vi "State Machine Kernel.vi"(4 "Init?":bool, 5 "Inputs":T4 {"Kobuki Sensors"."Charger Source" items=["DISCHARGING"=0, "DOCKING_CHARGED"=2, "DOCKING_CHARGING"=6, "ADAPTER_CHARGED"=18, "ADAPTER_CHARGING"=22]; "accelerometer"."z axis (g)" format="%.3f"; "accelerometer"."y axis (g)" format="%.3f"; "accelerometer"."x axis (g)" format="%.3f"}, 7 "StateData In":T1) -> (0 "Terminated?":bool, 2 "Outputs":T3, 3 "StateData Out":T1)   [LabVIEW 2017]
uses:
  controls/Inputs.ctl
  shared/Accelerometer.ctl
  Kobuki/KobukiSensors.ctl
  Kobuki/Kobuki Bumps and WheelDrops.ctl
  Kobuki/Kobuki Buttons.ctl
  controls/Outputs.ctl
  controls/StateData.ctl
  controls/StatesEnum.ctl
panel:
  # "Electrical: charging, battery, OI mode"
  # "Sensors: bump, cliff, button, wheel drop"
  # "Motors:"
  # "Inertia"
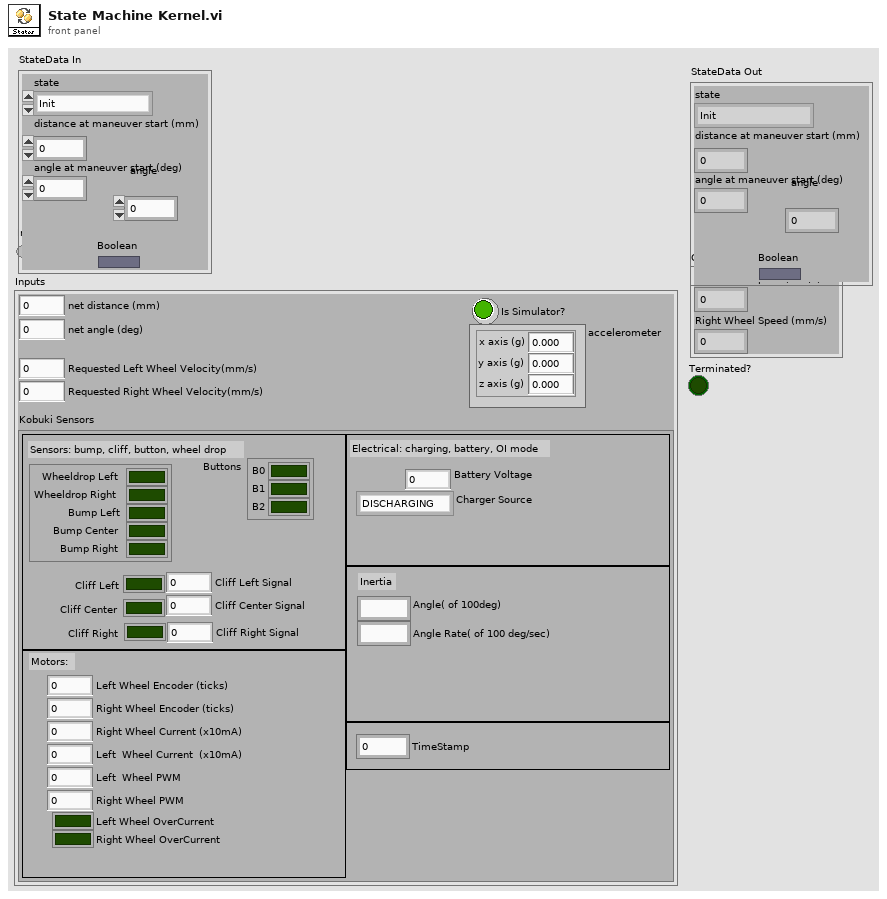
[diagram p1: front panel]
types:
  T1 = typedef "StateData.ctl" = cluster{"distance at maneuver start (mm)":i32, "angle at maneuver start (deg)":i32, "state":T2, "Boolean":bool, "angle":i32}
  T2 = typedef "StatesEnum.ctl" = enum16{"Init", "Center Cliff\n", "Pause", "Drive", "L.Cliff", "R.Cliff", "Shut"}
  T3 = typedef "Outputs.ctl" = cluster{"Left Wheel Speed (mm/s)":i16, "Right Wheel Speed (mm/s)":i16}
  T4 = typedef "Inputs.ctl" = cluster{"net distance (mm)":i32, "net angle (deg)":i32, "accelerometer":T5, "Is Simulator?":bool, "Kobuki Sensors":T6, "Requested Left Wheel Velocity(mm/s)":i32, "Requested Right Wheel Velocity(mm/s)":i32}
  T5 = typedef "Accelerometer.ctl" = cluster{"x axis (g)":dbl, "y axis (g)":dbl, "z axis (g)":dbl}
  T6 = typedef "KobukiSensors.ctl" = cluster{"Bumps + Wheel Drops":T7, "Cliff Left":bool, "Cliff Center":bool, "Cliff Right":bool, "Cliff Left Signal":u16, "Cliff Center Signal":u16, "Cliff Right Signal":u16, "Buttons":T8, "Left Wheel Encoder (ticks)":u16, "Right Wheel Encoder (ticks) ":u16, "Left  Wheel PWM":i8, "Right Wheel PWM":i8, "Left Wheel OverCurrent":bool, "Right Wheel OverCurrent ":bool, "Right Wheel Current (x10mA)":i16, "Left  Wheel Current  (x10mA)":i16, "TimeStamp":u16, "Battery Voltage":dbl, "Angle( of 100deg)":i16, "Angle Rate( of 100 deg/sec)":i16, "Charger Source ":i8}
  T7 = typedef "Kobuki Bumps and WheelDrops.ctl" = cluster{"Wheeldrop Left":bool, "Wheeldrop Right":bool, "Bump Left":bool, "Bump Center":bool, "Bump Right":bool}
  T8 = typedef "Kobuki Buttons.ctl" = cluster{"B0":bool, "B1":bool, "B2":bool}
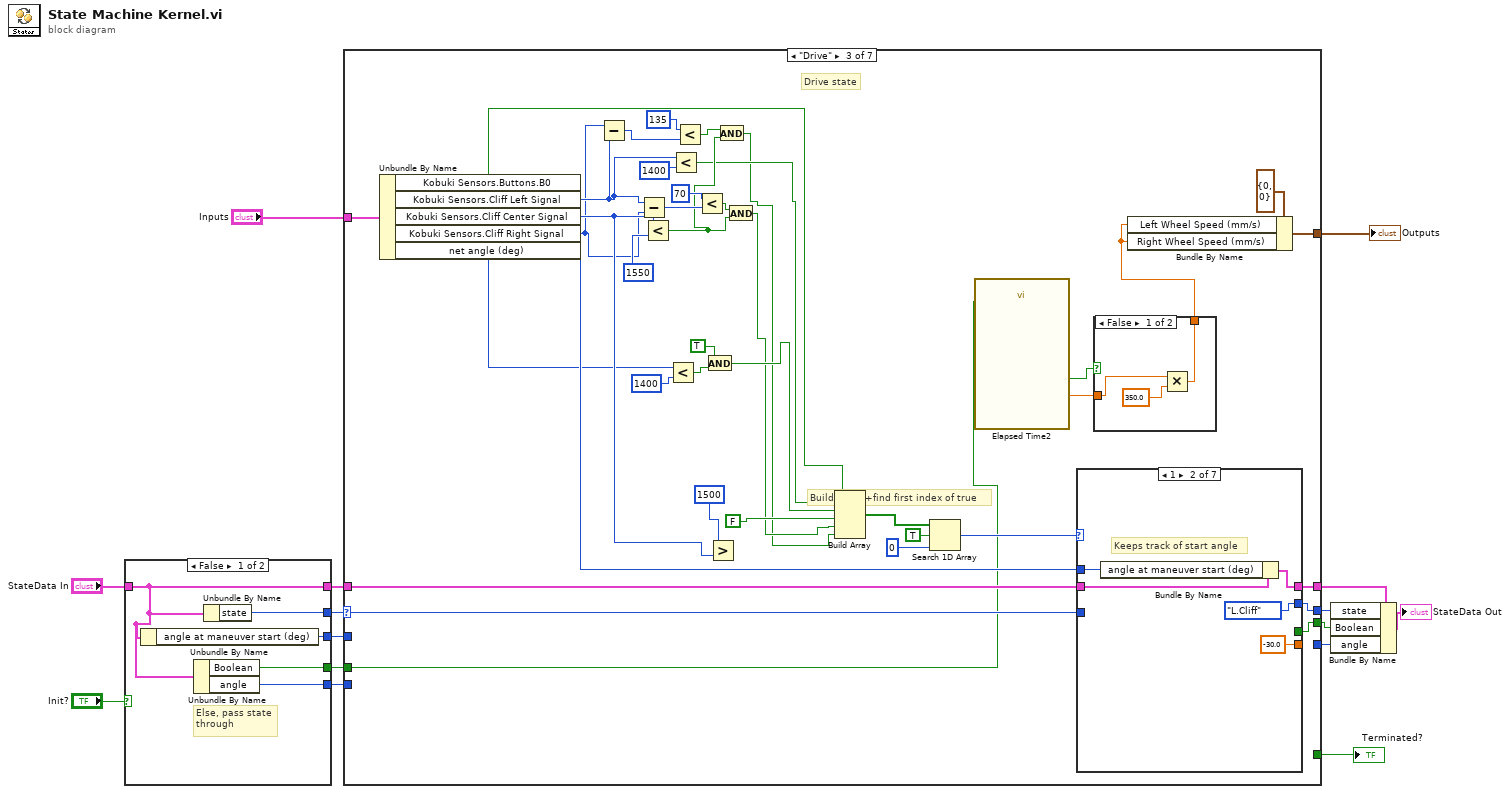
[diagram p0: block diagram]
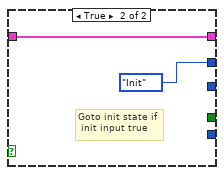
[diagram p2: hidden frame]
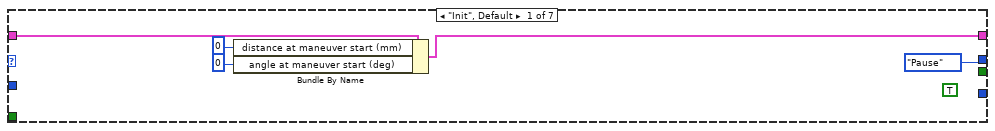
[diagram p3: hidden frame]
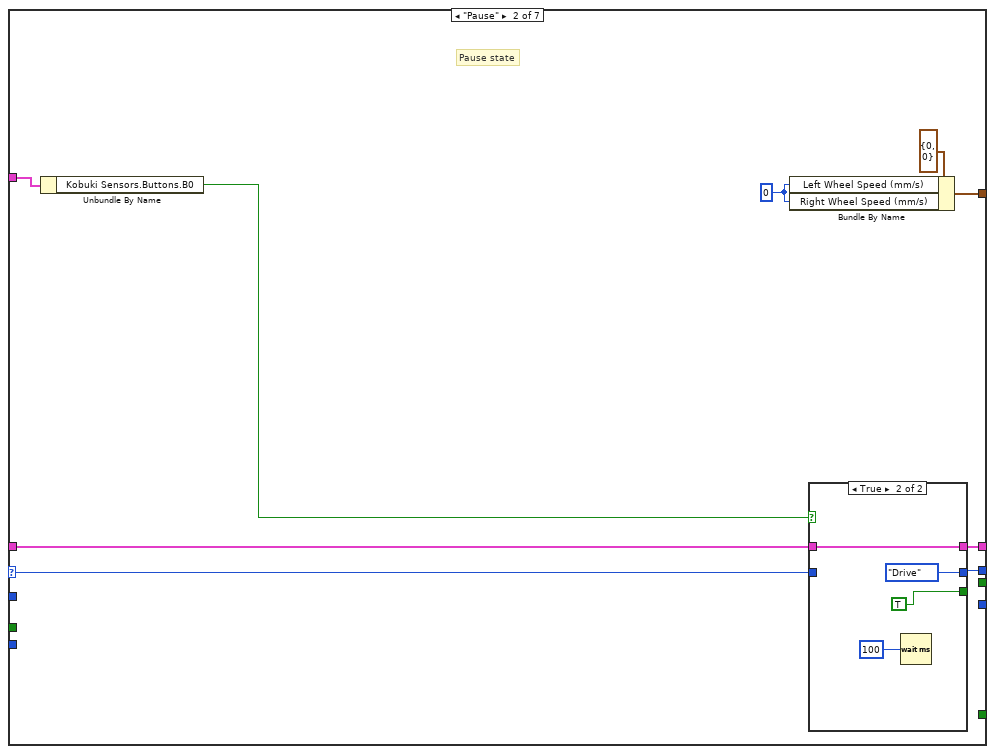
[diagram p4: hidden frame]
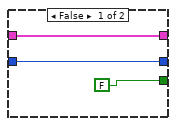
[diagram p5: hidden frame]
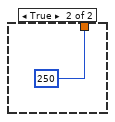
[diagram p6: hidden frame]
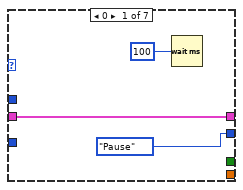
[diagram p7: hidden frame]
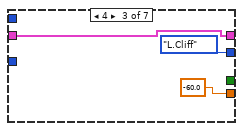
[diagram p8: hidden frame]
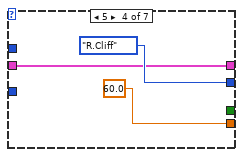
[diagram p9: hidden frame]
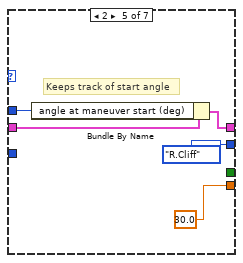
[diagram p10: hidden frame]
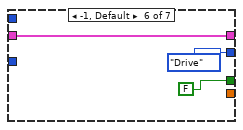
[diagram p11: hidden frame]
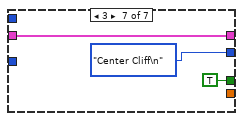
[diagram p12: hidden frame]
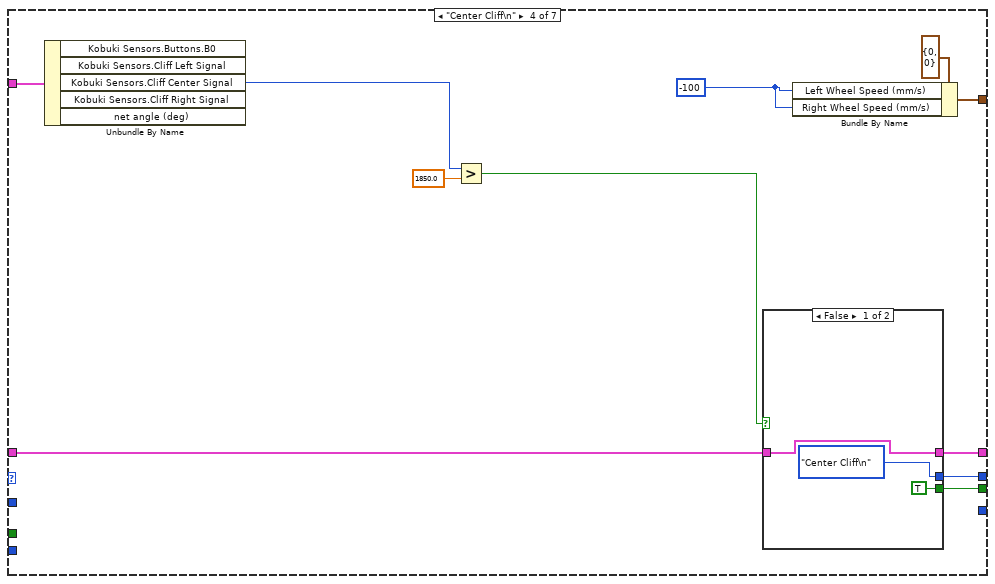
[diagram p13: hidden frame]
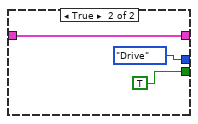
[diagram p14: hidden frame]
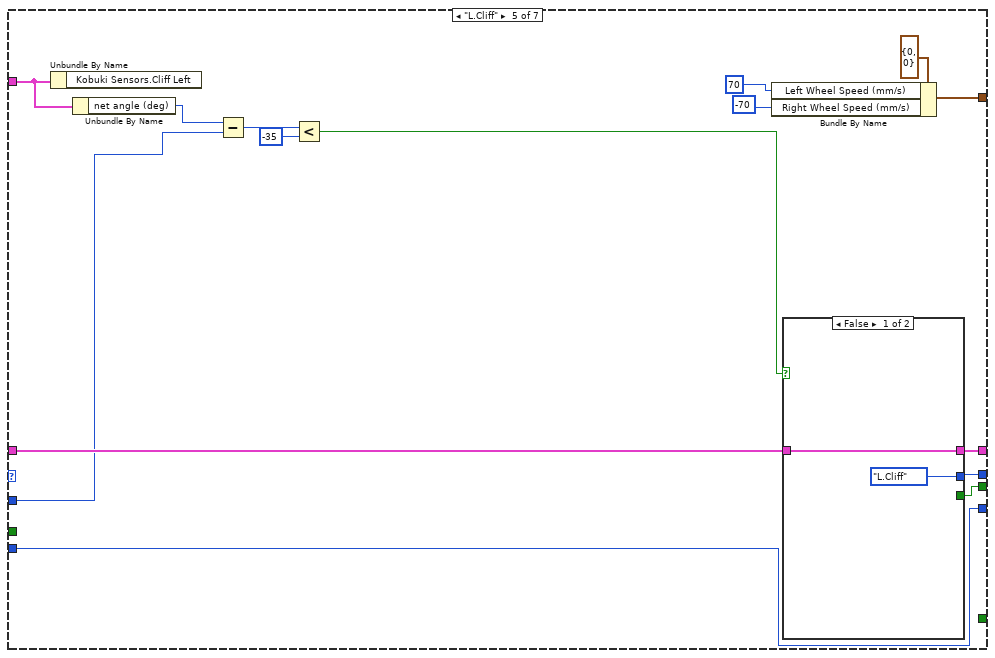
[diagram p15: hidden frame]
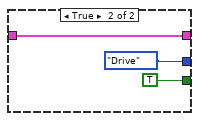
[diagram p16: hidden frame]
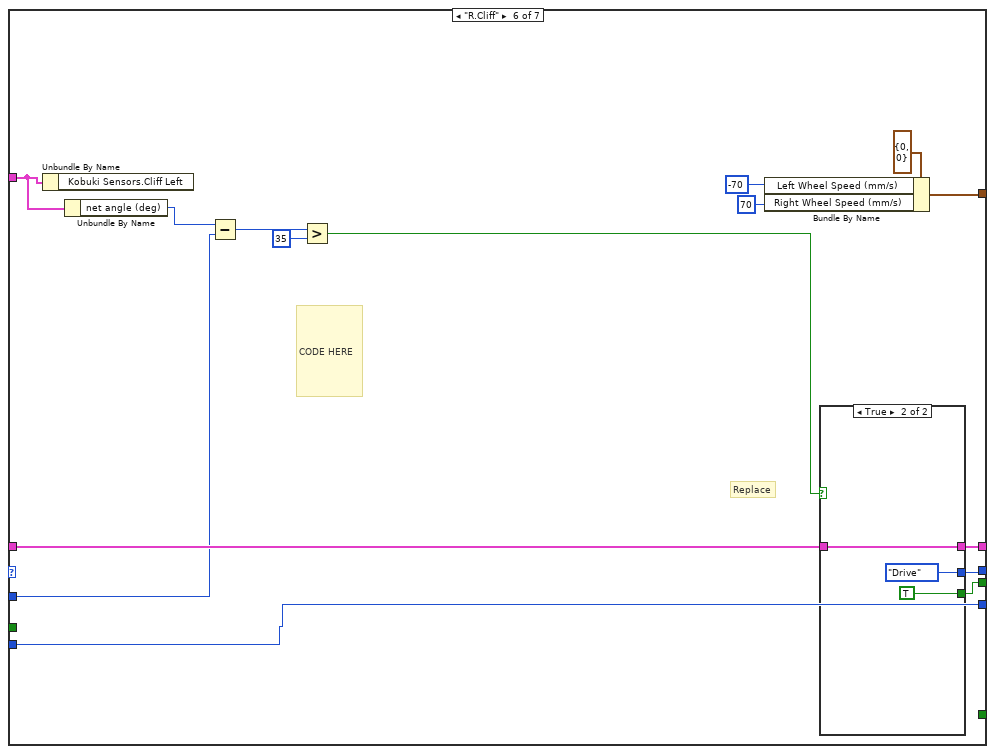
[diagram p17: hidden frame]
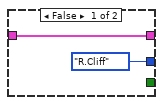
[diagram p18: hidden frame]
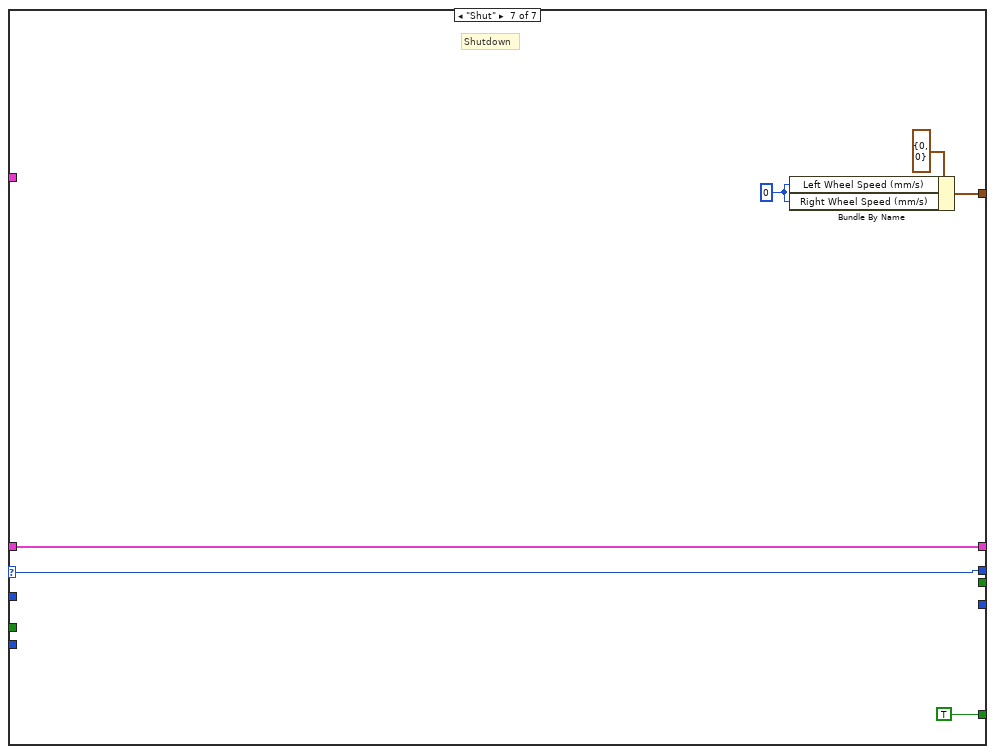
[diagram p19: hidden frame]
diagram:
  n1 = case shown="False" "Init?" {
    tunnel: [w20 StatesEnum."Init" ("StateIn")] -> w13
    tunnel: "StateData In" -> [w18 w21]
    tunnel: [w18 w21] -> w9
    tunnel: [w19 _] -> w6
    tunnel: [w17 _] -> w5
    tunnel: [w16 _] -> w2
    frame False {
      # "Else, pass state \nthrough"
      n2 = Unbundle By Name(w18) -> ("angle at maneuver start (deg)"=w19:i32)
      n3 = Unbundle By Name(w18) -> ("Boolean"=w17:bool, "angle"=w16:i32)
      n4 = Unbundle By Name(w18) -> ("state"=w20:T2)
    }
    frame True {
      # "Goto init state if\n init input true"
    }
  }
  n5 = case shown="\"Drive\"" w13 {
    selector: w13 -> [_ w32 w81 _ _ _ w169]
    tunnel: "Inputs" -> [_ w33 w82 w122 w139 w155 _]
    tunnel: [_ w36 w79 w120 w142 w160 w172] -> w11
    tunnel: [_ _ _ _ _ _ TRUE] -> w12
    tunnel: w9 -> [w27 w30 w74 w118 w140 w158 w170]
    tunnel: [w26 w29 w73 w117 w141 w159 w170] -> w8
    tunnel: w6 -> [_ _ _ _ w137 w154 _]
    tunnel: w5 -> [_ _ w67 _ _ _ _]
    tunnel: [_ _ w60 w116 w131 w151 _] -> w4
    tunnel: [StatesEnum."Pause" ("StateIn") w28 w61 w112 w132 w152 w169] -> w3
    tunnel: w2 -> [_ _ _ _ w130 w150 _]
    tunnel: [_ _ _ _ w130 w150 _] -> w1
    frame "Init", Default {
      (unwired) TRUE
      n6 = Bundle By Name(cluster=w27, "distance at maneuver start (mm)"=0, "angle at maneuver start (deg)"=0) -> (w26:T1)
    }
    frame "Pause" {
      w35 = i16 0 ("Left Wheel Speed (mm/s)")
      # "Pause state"
      n7 = Unbundle By Name(w33) -> ("Kobuki Sensors.Buttons.B0"=w34:bool)
      n8 = Bundle By Name(cluster=T3 {"Left Wheel Speed (mm/s)"=0, "Right Wheel Speed (mm/s)"=0} ("Outputs"), "Left Wheel Speed (mm/s)"=w35, "Right Wheel Speed (mm/s)"=w35) -> (w36:T3)
      n9 = case shown="True" w34 {
        tunnel: w32 -> [w39 _]
        tunnel: [w39 StatesEnum."Drive" ("StateIn")] -> w28
        tunnel: w30 -> [w38 w41]
        tunnel: [w38 w41] -> w29
        tunnel: [FALSE TRUE] -> _
        frame False {
        }
        frame True {
          n10 = Wait (ms)(milliseconds to wait=u32 100) -> ()  [unwired: 1 out]
        }
      }
    }
    frame "Drive" {
      # "Build array +find first index of true"
      # "Drive state"
      n11 = Unbundle By Name(w82) -> ("Kobuki Sensors.Buttons.B0"=w68:bool, "Kobuki Sensors.Cliff Left Signal"=w54:u16, "Kobuki Sensors.Cliff Center Signal"=w59:u16, "Kobuki Sensors.Cliff Right Signal"=w53:u16, "net angle (deg)"=w72:i32)
      n12 = Subtract(x=w53, y=w54) -> (x-y=w52:u16)
      n13 = Subtract(x=w54, y=w53) -> (x-y=w57:u16)
      n14 = Less?(x=w59, y=u16 1550) -> (x < y?=w50:bool)
      n15 = Less?(x=w53, y=u16 1400) -> (x < y?=w69:bool)
      n16 = Less?(x=w54, y=u16 1400) -> (x < y?=w47:bool)
      n17 = Less?(x=u16 135, y=w52) -> (x < y?=w49:bool)
      n18 = Less?(x=u16 70, y=w57) -> (x < y?=w55:bool)
      n19 = And(x=TRUE, y=w69) -> (x .and. y?=w48:bool)
      n20 = Greater?(x=u16 1500 ("y"), y=w59) -> ()  [unwired: 1 out]
      n21 = And(x=w49, y=w50) -> (x .and. y?=w44:bool)
      n22 = And(x=w55, y=w50) -> (x .and. y?=w45:bool)
      n23 = Build Array(w68, w47, w48, FALSE, w45, w44) -> (w78:bool[])
      n24 = Search 1D Array(1D array=w78, element=TRUE, start index (0)=0) -> (index of element=w75:i32)
      n25 = call "Elapsed Time2"("Reset"=w67) -> ("Elapsed Time (s)"=w65:dbl, "Time has Elapsed"=w66:bool)  [unwired: 11 in, 6 out]
      n26 = case shown="1" w75 {
        tunnel: w81 -> [_ _ _ _ _ _ _]
        tunnel: w74 -> [w88 w94 w95 w98 w105 w108 w110]
        tunnel: [w88 w92 w95 w98 w104 w108 w110] -> w73
        tunnel: w72 -> [_ w93 _ _ w103 _ _]
        tunnel: [_ _ _ _ _ FALSE TRUE] -> w60
        tunnel: [StatesEnum."Pause" ("StateIn") StatesEnum."L.Cliff" ("StateIn") StatesEnum."L.Cliff" ("StateIn") StatesEnum."R.Cliff" ("StateIn") StatesEnum."R.Cliff" ("StateIn") StatesEnum."Drive" ("StateIn") StatesEnum."Center Cliff\n" ("StateIn")] -> w61
        tunnel: [_ -30.0 ("angle") -60.0 ("angle") 60.0 ("angle") 30.0 ("angle") _ _] -> _
        frame 0 {
          n27 = Wait (ms)(milliseconds to wait=u32 100) -> ()  [unwired: 1 out]
        }
        frame 1 {
          # "Keeps track of start angle"
          n28 = Bundle By Name(cluster=w94, "angle at maneuver start (deg)"=w93) -> (w92:T1)
        }
        frame 4 {
        }
        frame 5 {
        }
        frame 2 {
          # "Keeps track of start angle"
          n29 = Bundle By Name(cluster=w105, "angle at maneuver start (deg)"=w103) -> (w104:T1)
        }
        frame -1, Default {
        }
        frame 3 {
        }
      }
      n30 = case shown="False" w66 {
        tunnel: w65 -> [w84 _]
        tunnel: [w83 250] -> w64
        frame False {
          n31 = Multiply(x=w84, y=350.0) -> (x*y=w83:dbl)
        }
        frame True {
        }
      }
      n32 = Bundle By Name(cluster=T3 {"Left Wheel Speed (mm/s)"=0, "Right Wheel Speed (mm/s)"=0} ("Outputs"), "Left Wheel Speed (mm/s)"=w64, "Right Wheel Speed (mm/s)"=w64) -> (w79:T3)
    }
    frame "Center Cliff\n" {
      w119 = i16 -100 ("Left Wheel Speed (mm/s)")
      n33 = Unbundle By Name(w122) -> ("Kobuki Sensors.Cliff Center Signal"=w114:u16)  [unwired: 4 out]
      n34 = Greater?(x=w114, y=1850.0) -> (0:w113:bool)
      n35 = case shown="False" w113 {
        tunnel: w118 -> [w124 w128]
        tunnel: [w124 w128] -> w117
        tunnel: [TRUE ("Boolean") TRUE ("Boolean")] -> w116
        tunnel: [StatesEnum."Center Cliff\n" ("StateIn") StatesEnum."Drive" ("StateIn")] -> w112
        frame False {
        }
        frame True {
        }
      }
      n36 = Bundle By Name(cluster=T3 {"Left Wheel Speed (mm/s)"=0, "Right Wheel Speed (mm/s)"=0} ("Outputs"), "Left Wheel Speed (mm/s)"=w119, "Right Wheel Speed (mm/s)"=w119) -> (w120:T3)
    }
    frame "L.Cliff" {
      n37 = Unbundle By Name(w139) -> ()  [unwired: 1 out]
      n38 = Unbundle By Name(w139) -> ("net angle (deg)"=w138:i32)
      n39 = Subtract(x=w138, y=w137) -> (x-y=w136:i32)
      n40 = Less?(x=w136, y=-35) -> (x < y?=w135:bool)
      n41 = Bundle By Name(cluster=T3 {"Left Wheel Speed (mm/s)"=0, "Right Wheel Speed (mm/s)"=0} ("Outputs"), "Left Wheel Speed (mm/s)"=i16 70 ("Right Wheel Speed (mm/s)"), "Right Wheel Speed (mm/s)"=i16 -70 ("Left Wheel Speed (mm/s)")) -> (w142:T3)
      n42 = case shown="False" w135 {
        tunnel: [StatesEnum."L.Cliff" ("StateIn") StatesEnum."Drive" ("StateIn")] -> w132
        tunnel: w140 -> [w144 w147]
        tunnel: [w144 w147] -> w141
        tunnel: [_ TRUE ("Boolean")] -> w131
        frame False {
        }
        frame True {
        }
      }
    }
    frame "R.Cliff" {
      # "Replace"
      # "CODE HERE"
      n43 = Unbundle By Name(w155) -> ()  [unwired: 1 out]
      n44 = Unbundle By Name(w155) -> ("net angle (deg)"=w156:i32)
      n45 = Subtract(x=w156, y=w154) -> (x-y=w157:i32)
      n46 = Greater?(x=w157, y=35) -> (0:w153:bool)
      n47 = Bundle By Name(cluster=T3 {"Left Wheel Speed (mm/s)"=0, "Right Wheel Speed (mm/s)"=0} ("Outputs"), "Left Wheel Speed (mm/s)"=i16 -70, "Right Wheel Speed (mm/s)"=i16 70) -> (w160:T3)
      n48 = case shown="True" w153 {
        tunnel: [StatesEnum."R.Cliff" ("StateIn") StatesEnum."Drive" ("StateIn")] -> w152
        tunnel: w158 -> [w164 w167]
        tunnel: [w164 w167] -> w159
        tunnel: [_ TRUE ("Boolean")] -> w151
        frame False {
        }
        frame True {
        }
      }
    }
    frame "Shut" {
      w173 = i16 0 ("Left Wheel Speed (mm/s)")
      # "Shutdown"
      n49 = Bundle By Name(cluster=T3 {"Left Wheel Speed (mm/s)"=0, "Right Wheel Speed (mm/s)"=0} ("Outputs"), "Left Wheel Speed (mm/s)"=w173, "Right Wheel Speed (mm/s)"=w173) -> (w172:T3)
    }
  }
  "Terminated?" <- w12
  "Outputs" <- w11
  n50 = Bundle By Name(cluster=w8, "state"=w3, "Boolean"=w4, "angle"=w1) -> (→"StateData Out":T1)
